vi "process.vi"(8 "error in (no error)":errorcluster, 11 "TCPConnectionHandler in":refnum<class "TCPConnectionHandler.lvclass">) -> (0 "error out":errorcluster, 3 "TCPConnectionHandler out":refnum<class "TCPConnectionHandler.lvclass">)   [LabVIEW 2013, in "MQTT Server.lvlib" / "TCPConnectionHandler.lvclass"]
uses:
  TCPConnectionHandler.lvclass
  TCPConnectionHandler.lvclass/TCPConnectionHandler.ctl
  Session/Session.lvclass
  Session/Session.lvclass/Session.ctl
  Connection/TCPConnection.lvclass
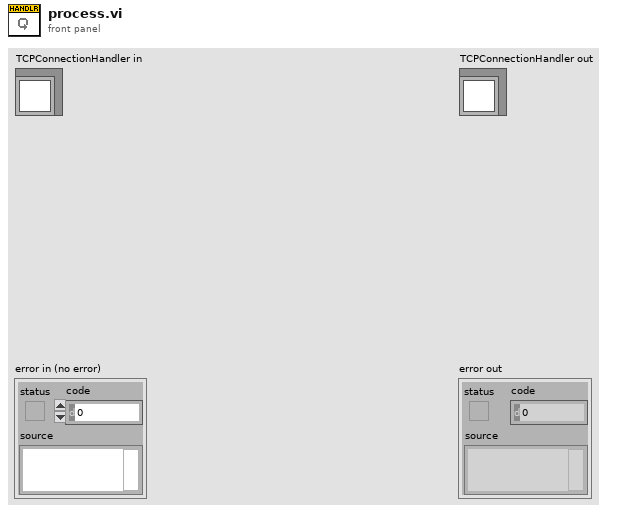
[diagram p1: front panel]
types:
  T1 = typedef "MQTT Server.lvlib/TCPConnectionHandler.lvclass/Private Events -- Cluster.ctl" = cluster{"Close Session Event":refnum<user-event>}
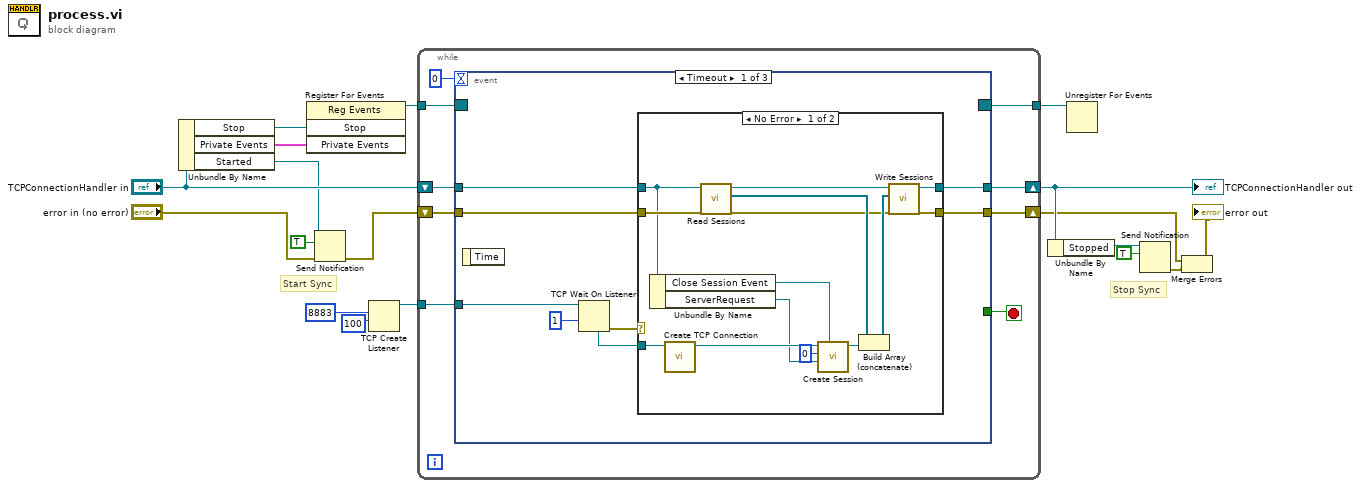
[diagram p0: block diagram]
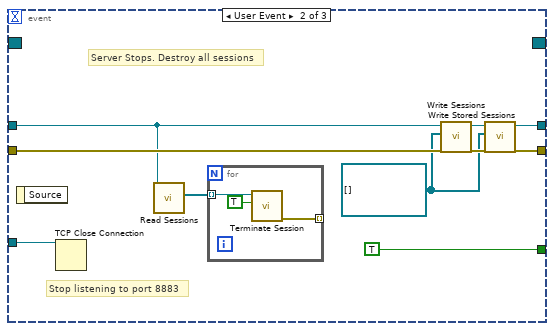
[diagram p3: hidden frame]
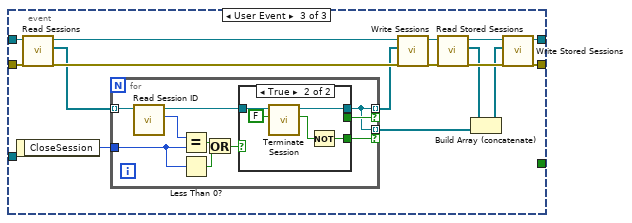
[diagram p4: hidden frame]
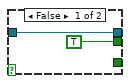
[diagram p5: hidden frame]
diagram:
  # "Stop Sync"
  # "Start Sync"
  n1 = Unbundle By Name("TCPConnectionHandler in") -> ("Stop"=w18:refnum<user-event>, "Private Events"=w11:T1, "Started"=w8:refnum<notifier>)
  n2 = register-events(w18, w11) -> (reference out=w13:refnum<event-registration>)  [unwired: 2 in, 1 out]
  n3 = Send Notification(notification=TRUE, notifier=w8, error in (no error)="error in (no error)") -> (error out=w9:errorcluster)  [unwired: 1 out]
  n4 = TCP Create Listener(9:100, 10:u16 8883 ("port")) -> (3:w16:refnum<k5>)  [unwired: 3 in, 2 out]
  n5 = while {
    shift-right: [w24] -> w7
    shift-left: "TCPConnectionHandler in" -> [w23]
    shift-right: [w26] -> w2
    shift-left: w9 -> [w25]
    tunnel: w13 -> [w22]
    tunnel: [w21] -> w17
    tunnel: w16 -> [w19]
    stop <- w20 stop-if-true
    n6 = event shown="[0] Timeout" {
      selector: w22 -> [_ _ _]
      dyn-events: [_ _ _] -> w21
      timeout: 0 -> [_ _ _]
      tunnel: [w28 w57 w72] -> w26
      tunnel: w25 -> [w30 w57 w72]
      tunnel: [w29 w51 w68] -> w24
      tunnel: w23 -> [w31 w54 w62]
      tunnel: [_ TRUE _] -> w20
      tunnel: w19 -> [w35 w53 _]
      event Timeout {
        n7 = event-data() -> ()  [unwired: 1 in, 1 out]
        n8 = TCP Wait On Listener(9:1, 11:w35) -> (0:w33:errorcluster, 4:w32:refnum<k5>)  [unwired: 2 in, 3 out]
        n9 = case shown="No Error" w33 {
          tunnel: w32 -> [w47 _]
          tunnel: w31 -> [w38 w49]
          tunnel: w30 -> [w40 w48]
          tunnel: [w39 w49] -> w29
          tunnel: [w40 w48] -> w28
          frame No Error {
            n10 = Unbundle By Name(w38) -> ("Close Session Event"=w36:refnum<user-event>, "ServerRequest"=w37:refnum<queue>)
            n11 = call "Create TCP Connection.vi"("connection ID"=w47) -> ("TCPConnection out"=w46:refnum<class "TCPConnection.lvclass">)  [unwired: 9 in, 1 out]
            n12 = call "Read Sessions.vi"("TCPConnectionHandler in"=w38) -> ("Sessions"=w42:refnum<class "Session.lvclass">[], "TCPConnectionHandler out"=w44:refnum<class "TCPConnectionHandler.lvclass">)  [unwired: 9 in]
            n13 = call "Create Session.vi"("Close Session"=w36, "ServerRequest"=w37, "Keep Alive (s)"=0, "Connection"=w46) -> ("Session"=w43:refnum<class "Session.lvclass">)  [unwired: 6 in, 1 out]
            n14 = Build Array (concatenate)(w42, w43) -> (w41:refnum<class "Session.lvclass">[])
            n15 = call "Write Sessions.vi"("Sessions"=w41, "TCPConnectionHandler in"=w44) -> ("TCPConnectionHandler out"=w39:refnum<class "TCPConnectionHandler.lvclass">)  [unwired: 9 in]
          }
          frame Error {
          }
        }
      }
      event User Event {
        w50 = refnum<class "Session.lvclass">[] [] ("Sessions")
        # "Stop listening to port 8883"
        # "Server Stops. Destroy all sessions"
        n16 = event-data() -> ()  [unwired: 1 in, 1 out]
        n17 = TCP Close Connection(connection ID=w53) -> ()  [unwired: 2 in, 2 out]
        n18 = call "Read Sessions.vi"("TCPConnectionHandler in"=w54) -> ("Sessions"=w55:refnum<class "Session.lvclass">[])  [unwired: 9 in, 1 out]
        n19 = for {
          tunnel: w55 -> [w60] mode=indexing
          tunnel: [w59] -> _ mode=indexing
          n20 = call "Terminate Session.vi"("Destroy (T)"=TRUE, "Session in"=w60) -> ("error out"=w59:errorcluster)  [unwired: 7 in, 2 out]
        }
        n21 = call "Write Sessions.vi"("Sessions"=w50, "TCPConnectionHandler in"=w54) -> ("TCPConnectionHandler out"=w52:refnum<class "TCPConnectionHandler.lvclass">)  [unwired: 9 in]
        n22 = call "Write Stored Sessions.vi"("Stored Sessions"=w50, "TCPConnectionHandler in"=w52) -> ("TCPConnectionHandler out"=w51:refnum<class "TCPConnectionHandler.lvclass">)  [unwired: 9 in]
      }
      event User Event {
        n23 = event-data() -> ("CloseSession"=w69:i32)  [unwired: 1 in]
        n24 = call "Read Sessions.vi"("TCPConnectionHandler in"=w62) -> ("Sessions"=w71:refnum<class "Session.lvclass">[], "TCPConnectionHandler out"=w61:refnum<class "TCPConnectionHandler.lvclass">)  [unwired: 9 in]
        n25 = for {
          tunnel: w71 -> [w81] mode=indexing
          tunnel: [w74] -> w70 mode=indexing if=w82
          tunnel: w69 -> [w76]
          tunnel: [w74] -> w64 mode=indexing if=w73
          n26 = call "Read Session ID.vi"("Session in"=w81) -> ("Session ID"=w79:i32, "Session out"=w80:refnum<class "Session.lvclass">)  [unwired: 8 in, 1 out]
          n27 = Equal?(x=w79, y=w76) -> (x = y?=w78:bool)
          n28 = Less Than 0?(x=w76) -> (x < 0?=w77:bool)
          n29 = Or(x=w78, y=w77) -> (x .or. y?=w75:bool)
          n30 = case shown="True" w75 {
            tunnel: w80 -> [w84 w89]
            tunnel: [w84 w88] -> w74
            tunnel: [TRUE _] -> w82
            tunnel: [_ w85] -> w73
            frame False {
            }
            frame True {
              n31 = call "Terminate Session.vi"("Destroy (T)"=FALSE, "Session in"=w89) -> ("Destroyed"=w86:bool, "Session out"=w88:refnum<class "Session.lvclass">)  [unwired: 7 in, 1 out]
              n32 = Not(x=w86) -> (.not. x?=w85:bool)
            }
          }
        }
        n33 = call "Write Sessions.vi"("Sessions"=w70, "TCPConnectionHandler in"=w61) -> ("TCPConnectionHandler out"=w67:refnum<class "TCPConnectionHandler.lvclass">)  [unwired: 9 in]
        n34 = call "Read Stored Sessions.vi"("TCPConnectionHandler in"=w67) -> ("Stored Sessions"=w65:refnum<class "Session.lvclass">[], "TCPConnectionHandler out"=w66:refnum<class "TCPConnectionHandler.lvclass">)  [unwired: 9 in]
        n35 = Build Array (concatenate)(w65, w64) -> (w63:refnum<class "Session.lvclass">[])
        n36 = call "Write Stored Sessions.vi"("Stored Sessions"=w63, "TCPConnectionHandler in"=w66) -> ("TCPConnectionHandler out"=w68:refnum<class "TCPConnectionHandler.lvclass">)  [unwired: 9 in]
      }
    }
  }
  "TCPConnectionHandler out" <- w7
  n37 = Unbundle By Name(w7) -> ("Stopped"=w6:refnum<notifier>)
  n38 = Unregister For Events(event registration refnum=w17) -> ()  [unwired: 1 in, 1 out]
  n39 = Send Notification(notification=TRUE, notifier=w6) -> (error out=w3:errorcluster)  [unwired: 1 in, 1 out]
  n40 = Merge Errors(w2, w3) -> (→"error out":errorcluster)
